vi "Manage Log File.vi"(8 "error in (no error)":errorcluster, 11 "LogRotate in":refnum<class "LogRotate.lvclass">) -> (0 "error out":errorcluster, 3 "LogRotate out":refnum<class "LogRotate.lvclass">)   [LabVIEW 2019, in "Error_Manager.lvlib" / "LogRotate.lvclass"]
uses:
  LogRotate.lvclass
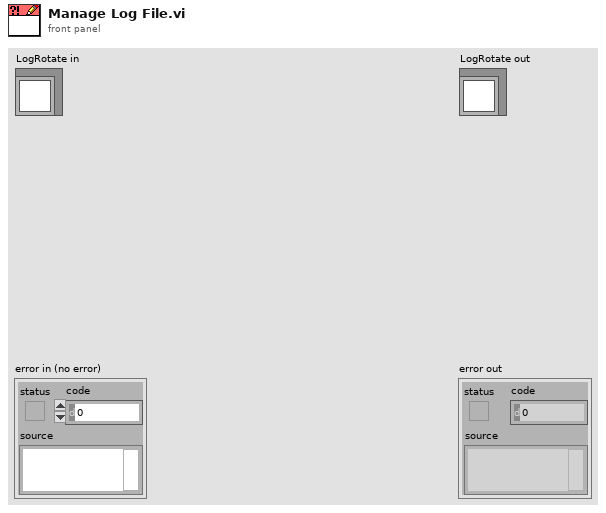
[diagram p1: front panel]
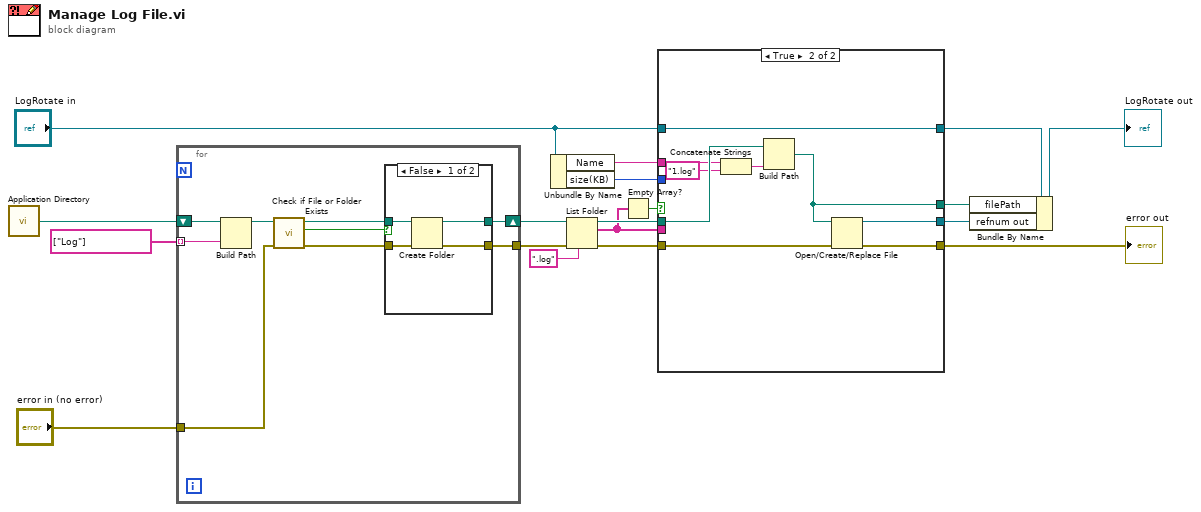
[diagram p0: block diagram]
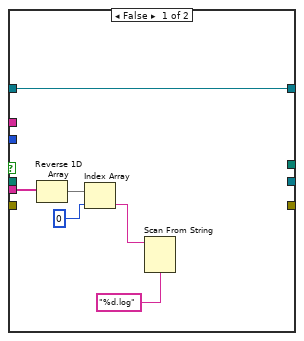
[diagram p2: hidden frame]
diagram:
  n1 = call <vilib>:"Application Directory.vi"() -> ("Application Directory"=w14:path)
  n2 = for {
    tunnel: string[] ["Log"] ("name or relative path") -> [w26] mode=indexing
    shift-right: [w21] -> w11
    shift-left: w14 -> [w27]
    tunnel: "error in (no error)" -> [w20]
    tunnel: [w19] -> w12
    n3 = Build Path(base path=w27, name or relative path=w26) -> (appended path=w25:path)
    n4 = call <vilib>:"Check if File or Folder Exists.vi"("error in (no error)"=w20, "path"=w25) -> ("error out"=w23:errorcluster, "file or folder exists?"=w24:bool, "dup path"=w22:path)  [unwired: 7 in]
    n5 = case shown="False" w24 {
      tunnel: w23 -> [w31 w32]
      tunnel: w22 -> [w30 w33]
      tunnel: [w29 w33] -> w21
      tunnel: [w28 w32] -> w19
      frame False {
        n6 = Create Folder(path (use dialog)=w30, error in=w31) -> (created path=w29:path, error out=w28:errorcluster)  [unwired: 1 in, 1 out]
      }
      frame True {
      }
    }
  }
  n7 = Unbundle By Name("LogRotate in") -> ("Name"=w5:string, "size(KB)"=w1:u32)
  n8 = List Folder(path=w11, pattern=".log", error in=w12) -> (path out=w7:path, filenames=w3:string[], error out=w9:errorcluster)  [unwired: 1 in, 1 out]
  n9 = Empty Array?(array=w3) -> (empty?=w8:bool)
  n10 = case shown="True" w8 {
    tunnel: w9 -> [_ w48]
    tunnel: [_ w47] -> w17
    tunnel: w7 -> [_ w46]
    tunnel: "LogRotate in" -> [w36 w45]
    tunnel: [w36 w45] -> w6
    tunnel: w5 -> [_ w44]
    tunnel: [_ w41] -> w4
    tunnel: w3 -> [w39 _]
    tunnel: [_ w40] -> w2
    tunnel: w1 -> [_ _]
    frame False {
      n11 = Reverse 1D Array(array=w39) -> (reversed array=w38:string[])
      n12 = Index Array(array=w38, index=0) -> (element=w35:string)
      n13 = Scan From String(format string="%d.log", input string=w35) -> ()  [unwired: 4 in, 3 out]
    }
    frame True {
      n14 = Concatenate Strings(w44, "1.log" ("string")) -> (w43:string)
      n15 = Build Path(base path=w46, name or relative path=w43) -> (appended path=w40:path)
      n16 = Open/Create/Replace File(file path (use dialog)=w40, error in=w48) -> (refnum out=w41:refnum<file>, error out=w47:errorcluster)  [unwired: 4 in, 1 out]
    }
  }
  "error out" <- w17
  n17 = Bundle By Name(cluster=w6, "filePath"=w2, "refnum out"=w4) -> (→"LogRotate out":refnum<class "LogRotate.lvclass">)
